vi "InitConfiguration.vi"(8 "error in":errorcluster) -> (0 "error out":errorcluster)   [LabVIEW 2013]
uses:
  <vilib>/Utility/config.llb/Read Key (U32).vi
  <vilib>/Utility/config.llb/Read Key (String).vi
  GlobalVariables/ValveParameters.vi
  <vilib>/Utility/config.llb/Read Key (Double).vi
  GlobalVariables/CaptParameters.vi
  GlobalVariables/SystemParameters.vi
  GlobalVariables/StabilizationSettings.vi
  <vilib>/Utility/config.llb/NI_LVConfig.lvlib
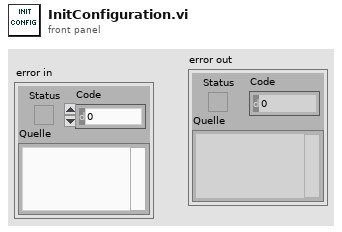
[diagram p1: front panel]
types:
  T1 = cluster{"Mode":enum16{"RTU", "ASCII"}, "Slave Address":u8}
  T2 = typedef "NI_LVConfig.lvlib/Config Data RefNum.ctl" = refnum<k1>
  T3 = cluster{"value":u32, "value":u32, "value":u32, "value":u32, "value":u32}
  T4 = cluster{"value":u32, "value":u32, "value":u32, "value":u32, "value":u32, "value":string, "Serial Parameters":cluster{"Mode":enum16{"RTU", "ASCII"}, "Slave Address":u8}, "value":u32, cluster{"value":u32, "value":u32, "value":u32, "value":u32, "value":u32}}
  T5 = cluster{"value":u32, "value":u32, "value":u32, "value":u32, "value":u32, "value":string, "value":u32, "Serial Parameters":cluster{"Mode":enum16{"RTU", "ASCII"}, "Slave Address":u8}, "value":u32, "value":dbl}
  T6 = cluster{"value":string, "value":string, "value":string, "value":string}
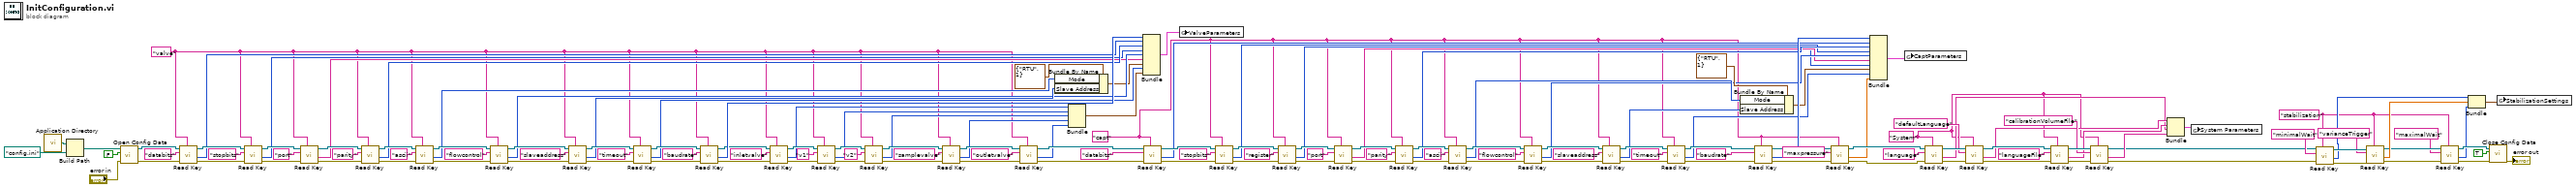
[diagram p0: block diagram]
diagram:
  w3 = "stabilization"
  w24 = "System" ("section")
  w12 = "capt" ("section")
  w30 = "valve" ("section")
  n1 = call <vilib>:"Application Directory.vi"() -> ("Application Directory"=w145:path)
  n2 = Build Path(base path=w145, name or relative path=path "config.ini" ("default name")) -> (appended path=w147:path)
  n3 = call <vilib>:"Open Config Data.vi"("error in (no error)"="error in", "create file if necessary (T)"=FALSE ("create file if necessary? (T)"), "configuration file path"=w147) -> ("error out"=w78:errorcluster, "refnum"=w77:T2)  [unwired: 6 in, 1 out]
  n4 = call-poly <vilib>:"Read Key.vi"("section"=w30, "error in (no error)"=w78, "key"="databits", "refnum"=w77) -> ("error out"=w81:errorcluster, "value"=w73:u32, "refnum out"=w80:T2)  [unwired: 4 in, 1 out]
  n5 = call-poly <vilib>:"Read Key.vi"("section"=w30, "error in (no error)"=w81, "key"="stopbits", "refnum"=w80) -> ("error out"=w79:errorcluster, "value"=w72:u32, "refnum out"=w76:T2)  [unwired: 4 in, 1 out]
  n6 = call-poly <vilib>:"Read Key.vi"("section"=w30, "error in (no error)"=w79, "key"="port", "refnum"=w76) -> ("error out"=w138:errorcluster, "value"=w118:string, "refnum out"=w137:T2)  [unwired: 4 in, 1 out]
  n7 = call-poly <vilib>:"Read Key.vi"("section"=w30, "error in (no error)"=w138, "key"="parity", "refnum"=w137) -> ("error out"=w135:errorcluster, "value"=w120:u32, "refnum out"=w132:T2)  [unwired: 4 in, 1 out]
  n8 = call-poly <vilib>:"Read Key.vi"("section"=w30, "error in (no error)"=w135, "key"="ascii", "refnum"=w132) -> ("error out"=w134:errorcluster, "value"=w125:u32, "refnum out"=w133:T2)  [unwired: 4 in, 1 out]
  n9 = call-poly <vilib>:"Read Key.vi"("section"=w30, "error in (no error)"=w134, "key"="flowcontrol", "refnum"=w133) -> ("error out"=w130:errorcluster, "value"=w119:u32, "refnum out"=w127:T2)  [unwired: 4 in, 1 out]
  n10 = call-poly <vilib>:"Read Key.vi"("section"=w30, "error in (no error)"=w130, "key"="slaveaddress", "refnum"=w127) -> ("error out"=w129:errorcluster, "value"=w124:u32, "refnum out"=w128:T2)  [unwired: 4 in, 1 out]
  n11 = call-poly <vilib>:"Read Key.vi"("section"=w30, "error in (no error)"=w129, "key"="timeout", "refnum"=w128) -> ("error out"=w142:errorcluster, "value"=w116:u32, "refnum out"=w143:T2)  [unwired: 4 in, 1 out]
  n12 = call-poly <vilib>:"Read Key.vi"("section"=w30, "error in (no error)"=w142, "key"="baudrate", "refnum"=w143) -> ("error out"=w47:errorcluster, "value"=w121:u32, "refnum out"=w37:T2)  [unwired: 4 in, 1 out]
  n13 = call-poly <vilib>:"Read Key.vi"("section"=w30, "error in (no error)"=w47, "key"="inletvalve", "refnum"=w37) -> ("error out"=w48:errorcluster, "value"=w35:u32, "refnum out"=w38:T2)  [unwired: 4 in, 1 out]
  n14 = call-poly <vilib>:"Read Key.vi"("section"=w30, "error in (no error)"=w48, "key"="v1", "refnum"=w38) -> ("error out"=w46:errorcluster, "value"=w34:u32, "refnum out"=w39:T2)  [unwired: 4 in, 1 out]
  n15 = call-poly <vilib>:"Read Key.vi"("section"=w30, "error in (no error)"=w46, "key"="v2", "refnum"=w39) -> ("error out"=w45:errorcluster, "value"=w33:u32, "refnum out"=w40:T2)  [unwired: 4 in, 1 out]
  n16 = call-poly <vilib>:"Read Key.vi"("section"=w30, "error in (no error)"=w45, "key"="samplevalve", "refnum"=w40) -> ("error out"=w44:errorcluster, "value"=w32:u32, "refnum out"=w41:T2)  [unwired: 4 in, 1 out]
  n17 = call-poly <vilib>:"Read Key.vi"("section"=w30, "error in (no error)"=w44, "key"="outletvalve", "refnum"=w41) -> ("error out"=w43:errorcluster, "value"=w31:u32, "refnum out"=w42:T2)  [unwired: 4 in, 1 out]
  n18 = Bundle By Name(cluster=T1 {"Mode"=enum."RTU", "Slave Address"=1} ("Serial Parameters"), "Mode"=w125, "Slave Address"=w124) -> (w117:T1)
  n19 = Bundle("value"=w35, "value"=w34, "value"=w33, "value"=w32, "value"=w31) -> (w36:T3)  [unwired: 1 in]
  n20 = Bundle("value"=w121, "value"=w73, "value"=w120, "value"=w72, "value"=w119, "value"=w118, "Serial Parameters"=w117, "value"=w116, w36) -> (w122:T4)  [unwired: 1 in]
  n21 = call-poly <vilib>:"Read Key.vi"("section"=w12, "error in (no error)"=w43, "key"="databits", "refnum"=w42) -> ("error out"=w71:errorcluster, "value"=w65:u32, "refnum out"=w70:T2)  [unwired: 4 in, 1 out]
  n22 = global write "ValveParameters.vi" "ValveParameters"(w122) -> ()
  n23 = call-poly <vilib>:"Read Key.vi"("section"=w12, "error in (no error)"=w71, "key"="stopbits", "refnum"=w70) -> ("error out"=w66:errorcluster, "value"=w64:u32, "refnum out"=w67:T2)  [unwired: 4 in, 1 out]
  n24 = call-poly <vilib>:"Read Key.vi"("section"=w12, "error in (no error)"=w66, "key"="register", "refnum"=w67) -> ("error out"=w85:errorcluster, "value"=w83:u32, "refnum out"=w84:T2)  [unwired: 4 in, 1 out]
  n25 = call-poly <vilib>:"Read Key.vi"("section"=w12, "error in (no error)"=w85, "key"="port", "refnum"=w84) -> ("error out"=w109:errorcluster, "value"=w90:string, "refnum out"=w108:T2)  [unwired: 4 in, 1 out]
  n26 = call-poly <vilib>:"Read Key.vi"("section"=w12, "error in (no error)"=w109, "key"="parity", "refnum"=w108) -> ("error out"=w106:errorcluster, "value"=w92:u32, "refnum out"=w103:T2)  [unwired: 4 in, 1 out]
  n27 = call-poly <vilib>:"Read Key.vi"("section"=w12, "error in (no error)"=w106, "key"="ascii", "refnum"=w103) -> ("error out"=w105:errorcluster, "value"=w96:u32, "refnum out"=w104:T2)  [unwired: 4 in, 1 out]
  n28 = call-poly <vilib>:"Read Key.vi"("section"=w12, "error in (no error)"=w105, "key"="flowcontrol", "refnum"=w104) -> ("error out"=w101:errorcluster, "value"=w91:u32, "refnum out"=w98:T2)  [unwired: 4 in, 1 out]
  n29 = call-poly <vilib>:"Read Key.vi"("section"=w12, "error in (no error)"=w101, "key"="slaveaddress", "refnum"=w98) -> ("error out"=w100:errorcluster, "value"=w95:u32, "refnum out"=w99:T2)  [unwired: 4 in, 1 out]
  n30 = call-poly <vilib>:"Read Key.vi"("section"=w12, "error in (no error)"=w100, "key"="timeout", "refnum"=w99) -> ("error out"=w112:errorcluster, "value"=w88:u32, "refnum out"=w113:T2)  [unwired: 4 in, 1 out]
  n31 = Bundle By Name(cluster=T1 {"Mode"=enum."RTU", "Slave Address"=1} ("Serial Parameters"), "Mode"=w96, "Slave Address"=w95) -> (w89:T1)
  n32 = call-poly <vilib>:"Read Key.vi"("section"=w12, "error in (no error)"=w112, "key"="baudrate", "refnum"=w113) -> ("error out"=w16:errorcluster, "value"=w93:u32, "refnum out"=w14:T2)  [unwired: 4 in, 1 out]
  n33 = call-poly <vilib>:"Read Key.vi"("section"=w12, "error in (no error)"=w16, "key"="maxpressure", "refnum"=w14) -> ("error out"=w15:errorcluster, "value"=w10:dbl, "refnum out"=w13:T2)  [unwired: 4 in, 1 out]
  n34 = Bundle("value"=w93, "value"=w65, "value"=w92, "value"=w64, "value"=w91, "value"=w90, "value"=w83, "Serial Parameters"=w89, "value"=w88, "value"=w10) -> (w86:T5)  [unwired: 1 in]
  n35 = global write "CaptParameters.vi" "CaptParameters"(w86) -> ()
  n36 = call-poly <vilib>:"Read Key.vi"("section"=w24, "error in (no error)"=w15, "key"="language" ("section"), "refnum"=w13) -> ("error out"=w58:errorcluster, "value"=w51:string, "refnum out"=w63:T2)  [unwired: 4 in, 1 out]
  n37 = call-poly <vilib>:"Read Key.vi"("section"=w24, "error in (no error)"=w58, "key"="defaultLanguage" ("section"), "refnum"=w63) -> ("error out"=w59:errorcluster, "value"=w53:string, "refnum out"=w62:T2)  [unwired: 4 in, 1 out]
  n38 = call-poly <vilib>:"Read Key.vi"("section"=w24, "error in (no error)"=w59, "key"="languageFile" ("section"), "refnum"=w62) -> ("error out"=w60:errorcluster, "value"=w52:string, "refnum out"=w61:T2)  [unwired: 4 in, 1 out]
  n39 = call-poly <vilib>:"Read Key.vi"("section"=w24, "error in (no error)"=w60, "key"="calibrationVolumeFile" ("section"), "refnum"=w61) -> ("error out"=w9:errorcluster, "value"=w50:string, "refnum out"=w8:T2)  [unwired: 4 in, 1 out]
  n40 = Bundle("value"=w53, "value"=w52, "value"=w51, "value"=w50) -> (w49:T6)  [unwired: 1 in]
  n41 = global write "SystemParameters.vi" "System Parameters"(w49) -> ()
  n42 = call-poly <vilib>:"Read Key.vi"("section"=w3, "error in (no error)"=w9, "key"="minimalWait", "refnum"=w8) -> ("error out"=w23:errorcluster, "value"=w18:u32, "refnum out"=w22:T2)  [unwired: 4 in, 1 out]
  n43 = call-poly <vilib>:"Read Key.vi"("section"=w3, "error in (no error)"=w23, "key"="varianceTrigger", "refnum"=w22) -> ("error out"=w4:errorcluster, "value"=w17:dbl, "refnum out"=w7:T2)  [unwired: 4 in, 1 out]
  n44 = call-poly <vilib>:"Read Key.vi"("section"=w3, "error in (no error)"=w4, "key"="maximalWait", "refnum"=w7) -> ("error out"=w5:errorcluster, "value"=w1:u32, "refnum out"=w6:T2)  [unwired: 4 in, 1 out]
  n45 = Bundle("value"=w18, "value"=w17, "value"=w1) -> (w19:cluster{"value":u32, "value":dbl, "value":u32})  [unwired: 1 in]
  n46 = call <vilib>:"Close Config Data.vi"("error in (no error)"=w5, "write file if changed (T)"=TRUE ("write configuration file? (T)"), "refnum"=w6) -> ("error out"=→"error out":errorcluster)  [unwired: 8 out]
  n47 = global write "StabilizationSettings.vi" "StabilizationSettings"(w19) -> ()
